vi "EOMscan.vi"() -> ()   [LabVIEW 2011]
uses:
  <vilib>/DAQmx/write.llb/DAQmx Write (Analog DBL 1Chan 1Samp).vi
  <vilib>/DAQmx/read.llb/DAQmx Read (Analog DBL 1Chan 1Samp).vi
  <vilib>/DAQmx/create/channels.llb/DAQmx Create Channel (AO-Voltage-Basic).vi
  <vilib>/DAQmx/create/channels.llb/DAQmx Create Channel (AI-Voltage-Basic).vi
  <vilib>/DAQmx/miscellaneous.llb/DAQmx Fill In Error Info.vi
  <vilib>/Utility/file.llb/Write To Spreadsheet File (DBL).vi
  <vilib>/Analysis/NI_AAL_SigProc.lvlib
panel:
  in  "Use diode\nlinerarization":bool=TRUE
  in  "photodiode in":tag="Dev2/ai0"
  in  "EOM out ch":tag="Dev2/ao0"
  out "Maxima":dbl=4.420695186351812
  out "Minima at V":dbl=1.326353835924355
  in  "Save ascii after run":bool
  out "EOM - PD":cluster{dbl[], dbl[]}(graph)
  out "PhotoDiode":dbl=0.8774483613041534 format="%.5f"
  out "Actual U-out":dbl=4.983333333333333
  in  "Steps":u16=300
  in  "Umax":dbl=5.0
  # "1024 is ok\n4096 ia AD-sampler"
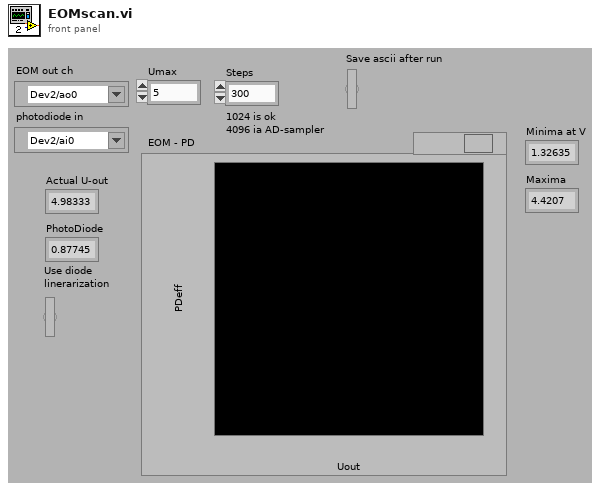
[diagram p1: front panel]
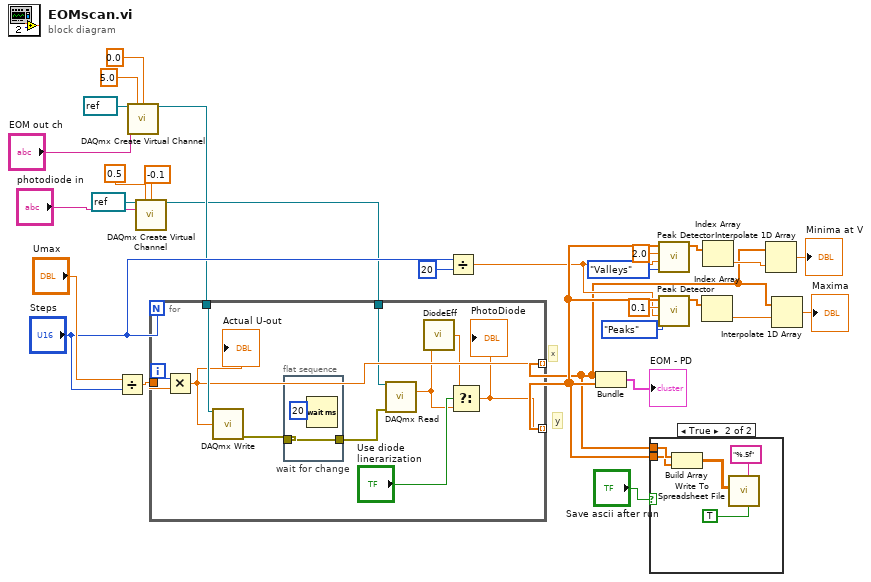
[diagram p0: block diagram]
diagram:
  # "y"
  # "x"
  n1 = Divide(x="Umax", y="Steps") -> (x/y=w28:dbl)
  n2 = call-poly <vilib>:"DAQmx Create Virtual Channel.vi"("task in"=refnum<k21> refnum, "maximum value"=5.0, "minimum value"=0.0, "physical channels"="EOM out ch") -> ("task out"=w2:refnum<k21>)  [unwired: 5 in, 6 out]
  n3 = call-poly <vilib>:"DAQmx Create Virtual Channel.vi"("task in"=refnum<k21> refnum, "maximum value"=0.5, "minimum value"=-0.1, "physical channels"="photodiode in") -> ("task out"=w1:refnum<k21>)  [unwired: 5 in, 6 out]
  n4 = for {
    N: "Steps" -> [_]
    tunnel: w28 -> [w39]
    tunnel: [w37] -> w12 mode=indexing
    tunnel: [w31] -> w18 mode=indexing
    tunnel: w2 -> [w38]
    tunnel: w1 -> [w34]
    i -> [w40]
    n5 = Multiply(x=w40, y=w39) -> (x*y=w37:dbl)
    "Actual U-out" <- w37
    n6 = call-poly <vilib>:"DAQmx Write.vi"("task/channels in"=w38, "data"=w37) -> ("error out"=w36:errorcluster)  [unwired: 2 in, 11 out]
    n7 = flat-sequence "wait for change" {
      tunnel: w36 -> [w42]
      tunnel: [w42] -> w35
      frame #0 {
        n8 = Wait (ms)(milliseconds to wait=u32 20) -> ()  [unwired: 1 out]
      }
    }
    n9 = call-poly <vilib>:"DAQmx Read.vi"("task/channels in"=w34, "error in"=w35) -> ("data"=w30:dbl)  [unwired: 13 out]
    n10 = call "DiodeEff.vi"("DiodeU"=w30) -> ("DiodeUeff"=w32:dbl)
    n11 = Select(t=w32, s="Use diode\nlinerarization", f=w30) -> (s? t:f=w31:dbl)
    "PhotoDiode" <- w31
  }
  n12 = Divide(x="Steps", y=u16 20) -> (x/y=w15:dbl)
  n13 = Bundle(w12, w18) -> (→"EOM - PD":cluster{dbl[], dbl[]})  [unwired: 1 in]
  n14 = case shown="True" "Save ascii after run" {
    tunnel: w12 -> [_ w47]
    tunnel: w18 -> [_ w46]
    frame False {
    }
    frame True {
      n15 = Build Array(w47, w46) -> (w45:dbl[][])
      n16 = call-poly <vilib>:"Write To Spreadsheet File.vi"("transpose? (no:F)"=TRUE, "format (%.3f)"="%.5f", "2D data"=w45) -> ()  [unwired: 5 in, 1 out]
    }
  }
  n17 = call <vilib>:"Peak Detector.vi"("peaks/valleys"=enum32{"Peaks", "Valleys"}."Valleys", "width"=w15, "threshold"=2.0, "X"=w18) -> ("Locations"=w21:dbl[])  [unwired: 3 in, 4 out]
  n18 = call <vilib>:"Peak Detector.vi"("peaks/valleys"=enum32{"Peaks", "Valleys"}."Peaks", "width"=w15, "threshold"=0.1, "X"=w18) -> ("Locations"=w14:dbl[])  [unwired: 3 in, 4 out]
  n19 = Index Array(array=w14) -> (element=w13:dbl)  [unwired: 1 in]
  n20 = Index Array(array=w21) -> (element=w20:dbl)  [unwired: 1 in]
  n21 = Interpolate 1D Array(1:w20, 2:w12) -> (0:→"Minima at V":dbl)
  n22 = Interpolate 1D Array(1:w13, 2:w12) -> (0:→"Maxima":dbl)
